vi "Write Blackboard.vi"(8 "error in (no error)":errorcluster, 10 "BT.lvlib:bt_Blackboard.lvclass":refnum<class "bt_Blackboard.lvclass">, 11 "bt_System in":refnum<class "bt_System.lvclass">) -> (0 "error out":errorcluster, 3 "bt_System out":refnum<class "bt_System.lvclass">)   [LabVIEW 2021, in "BT.lvlib" / "bt_System.lvclass"]
uses:
  bt_System.lvclass
  bt_System.lvclass/bt_System.ctl
  Blackboard/bt_Blackboard.lvclass
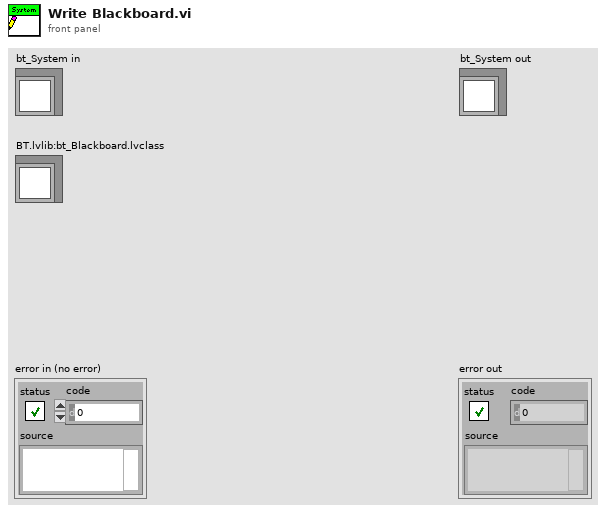
[diagram p1: front panel]
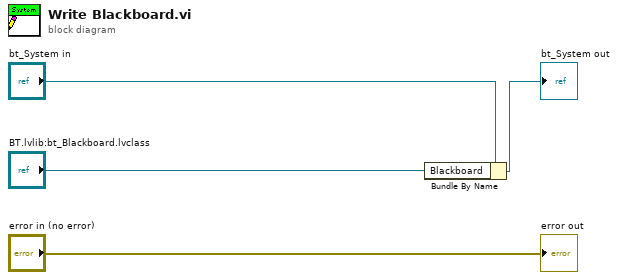
[diagram p0: block diagram]
diagram:
  n1 = Bundle By Name(cluster="bt_System in", "Blackboard"="BT.lvlib:bt_Blackboard.lvclass") -> (→"bt_System out":refnum<class "bt_System.lvclass">)
  "error out" <- "error in (no error)"
